vi "fg_references.vi"(7 "command":T3=enum."read", 8 "error in (no error)":errorcluster, 11 "references in":T1) -> (0 "error out":errorcluster, 3 "references out":T1)   [LabVIEW 2015, in "lv-recipe-machine.lvlib"]
uses:
  lv-recipe-machine.lvlib
  _controls/references.ctl
  public/_controls/input.ctl
  _controls/input_command.ctl
  _controls/output.ctl
  public/_controls/transition.ctl
  _controls/data.ctl
  public/_controls/configuration.ctl
  _controls/recipe_data.ctl
  public/_controls/mode.ctl
  public/_controls/manual_state.ctl
  public/_controls/automatic_state.ctl
  _controls/timer.ctl
  public/_controls/recipe_step.ctl
  public/_controls/change.ctl
  public/_controls/status.ctl
  _controls/fg_command.ctl
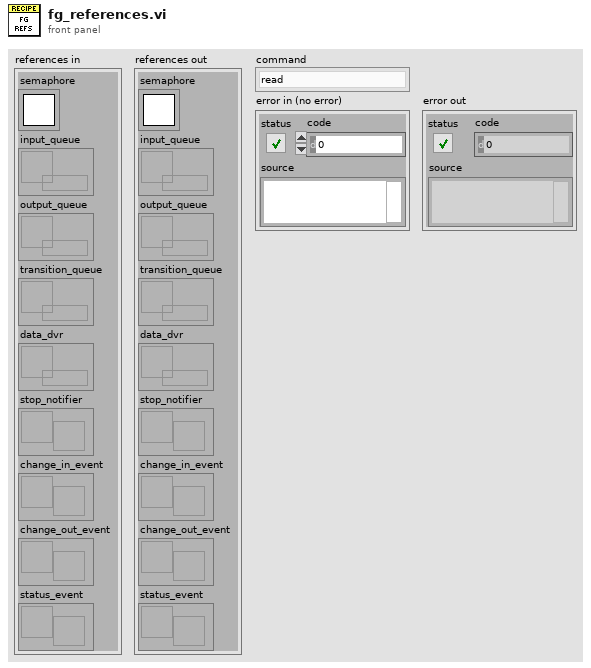
[diagram p1: front panel]
types:
  T1 = typedef "lv-recipe-machine.lvlib/references.ctl" = cluster{"semaphore":T2, "input_queue":refnum<queue>, "output_queue":refnum<queue>, "transition_queue":refnum<queue>, "data_dvr":refnum<data-value>, "stop_notifier":refnum<notifier>, "change_in_event":refnum<user-event>, "change_out_event":refnum<user-event>, "status_event":refnum<user-event>}
  T2 = typedef "Semaphore RefNum" = refnum<k1>
  T3 = typedef "lv-recipe-machine.lvlib/fg_command.ctl" = enum16{"<fg_command>", "initialize", "read", "write", "shutdown", "<null>"}
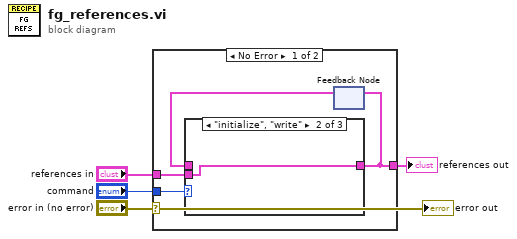
[diagram p0: block diagram]
diagram:
  n1 = case shown="No Error" "error in (no error)" {
    tunnel: "command" -> [w8 _]
    tunnel: "references in" -> [w7 _]
    tunnel: [w5 _] -> w1
    frame No Error {
      n2 = feedback #1() -> (w6:T1)  [unwired: 1 in]
      n3 = case shown="\"initialize\", \"write\"" w8 {
        tunnel: w7 -> [_ w10 _]
        tunnel: [w9 w10 _] -> w5
        tunnel: w6 -> [w9 _ _]
        frame Default {
        }
        frame "initialize", "write" {
        }
        frame "shutdown" {
        }
      }
      n4 = feedback-in #1(w5) -> ()
    }
    frame Error {
    }
  }
  "references out" <- w1
  "error out" <- "error in (no error)"
